vi "calculator.vi"() -> ()   [LabVIEW 2023]
panel:
  in  "stop":bool
  out "c":dbl
  in  "div":bool
  in  "mul":bool
  in  "sub":bool
  in  "add":bool
  in  "b":dbl
  in  "a":dbl
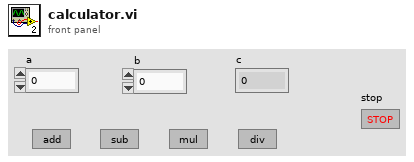
[diagram p1: front panel]
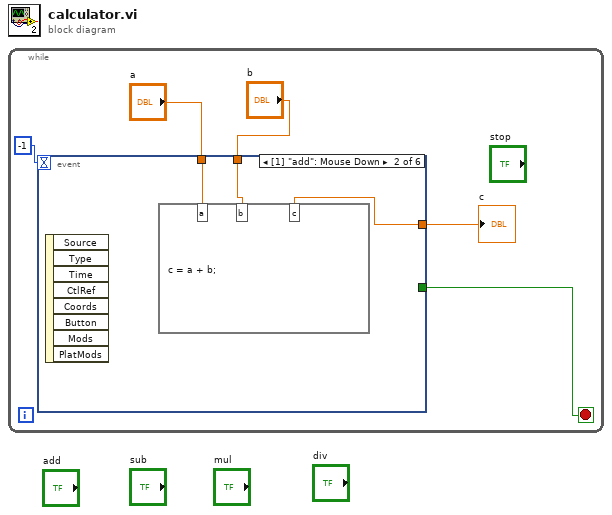
[diagram p0: block diagram]
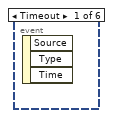
[diagram p2: hidden frame]
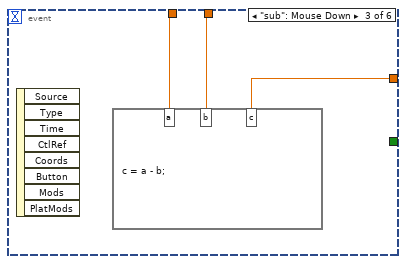
[diagram p3: hidden frame]
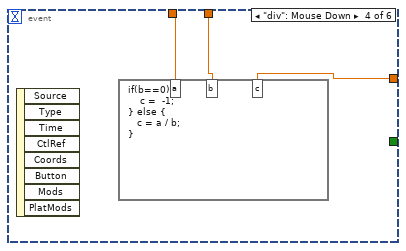
[diagram p4: hidden frame]
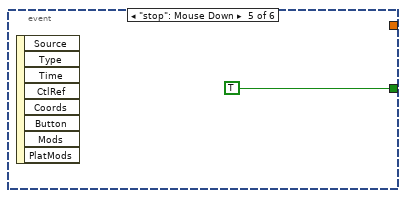
[diagram p5: hidden frame]
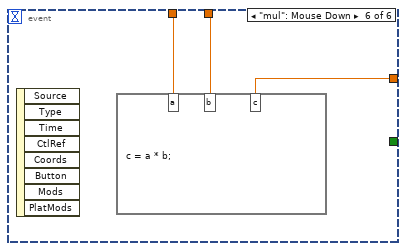
[diagram p6: hidden frame]
diagram:
  n1 = while {
    stop <- w1 stop-if-true
    n2 = event shown="[1] \"add\": Mouse Down" {
      selector: _ -> [_ _ _ _ _ _]
      dyn-events: _ -> [_ _ _ _ _ _]
      timeout: -1 -> [_ _ _ _ _ _]
      tunnel: "a" -> [_ w8 w11 w14 _ w18]
      tunnel: "b" -> [_ w7 w10 w13 _ w17]
      tunnel: [_ w6 w9 w12 _ w16] -> w2
      tunnel: [_ _ _ _ TRUE _] -> w1
      event Timeout {
        n3 = event-data() -> ()  [unwired: 1 in, 3 out]
      }
      event "add": Mouse Down {
        n4 = event-data() -> ()  [unwired: 1 in, 8 out]
        n5 = formula code="c = a + b;"("a"=w8, "b"=w7) -> ("c"=w6:dbl)
      }
      event "sub": Mouse Down {
        n6 = event-data() -> ()  [unwired: 1 in, 8 out]
        n7 = formula code="c = a - b;"("a"=w11, "b"=w10) -> ("c"=w9:dbl)
      }
      event "div": Mouse Down {
        n8 = event-data() -> ()  [unwired: 1 in, 8 out]
        n9 = formula code="if(b==0)  {\n    c =  -1;\n} else {\n   c = a / b;\n}"("a"=w14, "b"=w13) -> ("c"=w12:dbl)
      }
      event "stop": Mouse Down {
        n10 = event-data() -> ()  [unwired: 1 in, 8 out]
      }
      event "mul": Mouse Down {
        n11 = event-data() -> ()  [unwired: 1 in, 8 out]
        n12 = formula code="c = a * b;"("a"=w18, "b"=w17) -> ("c"=w16:dbl)
      }
    }
    "c" <- w2
  }
